vi "Load-default-advanced-params-from-file.vi"(8 "error in":errorcluster, 11 "Data ref. in":refnum<data-value>) -> (0 "error IO":errorcluster, 3 "Data ref.":refnum<data-value>)   [LabVIEW 2013, in "CameraVision.lvlib" / "CV-Main.lvclass"]
doc: "This function loads the default values for the hidden program parameters from an .xml file and writes these values to the parameter groups.\nThe file path for the hidden parameters is '<Application directory>\\Program data\\parameters-hidden.xml'.\nThe hidden parameters can not be changed through the CameraVision program, but can be changed using the 'CV-Set-hidden-parameters.vi' utility."
uses:
  CV-Main.lvclass
  Parameters-advanced.ctl
  Configuration/Configuration-parameters-advanced.ctl
  Acquisition/Acquisition-parameters-advanced.ctl
  Correction/Correction-parameters-advanced.ctl
  Analysis/Analysis-parameters-advanced.ctl
  Temperature/Temperature-parameters-advanced.ctl
  Storage/Storage-parameters-advanced.ctl
  Storage/Storage-types-labels.ctl
  CV-Main.lvclass/CV-Main.ctl
  Read Config params.vi
  Read Acquis params.vi
  Read Storage params.vi
  Read Correct params.vi
  Read Analysis params.vi
  Read Temperature params.vi
  <vilib>/Utility/xml.llb/Read From XML File(string).vi
  Temperature/Overwrite-all-hidden-params.vi
  Analysis/Overwrite-all-hidden-parameters.vi
  Correction/Overwrite-all-hidden-params.vi
  Storage/Overwrite-all-hidden-params.vi
  Acquisition/Overwrite-all-hidden-parameters.vi
  Configuration/Overwrite-all-hidden-params.vi
  Configuration/CV-Configuration.lvclass
  Acquisition/CV-Acquisition.lvclass
  Storage/CV-Storage.lvclass
  Correction/CV-Correction.lvclass
  Analysis/CV-Analysis.lvclass
  Temperature/CV-Temperature.lvclass
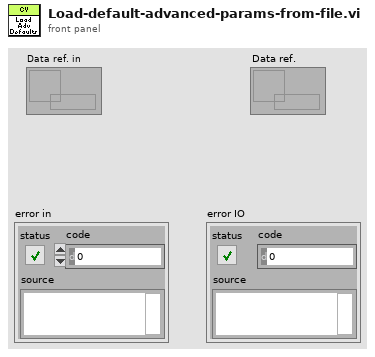
[diagram p1: front panel]
types:
  T1 = typedef "CameraVision.lvlib/CV-Main.lvclass/Parameters-advanced.ctl" = cluster{"Config params adv":T2, "Acquis params adv":T3, "Correct params adv":T4, "Analys params adv":T5, "Temp params adv":T7, "Storage params adv":T8}
  T2 = typedef "CameraVision.lvlib/CV-Configuration.lvclass/Configuration-parameters-advanced.ctl" = cluster{"Image border size":i32, "Framegrabber board":i32, "Framegrabber buffer":i32, "Camera config file":path, "Framegrabber DLL file":path}
  T3 = typedef "CameraVision.lvlib/CV-Acquisition.lvclass/Acquisition-parameters-advanced.ctl" = cluster{"Image acquisition timeout factor":dbl, "Image collection timeout factor":dbl, "Manual trigger ID":u8, "Precision hardware counter":tag, "When to use gate signal?":bool, "Minimum acquisition timeout":i32, "External timing channel":tag, "External gating channel":tag}
  T4 = typedef "CameraVision.lvlib/CV-Correction.lvclass/Correction-parameters-advanced.ctl" = cluster{"2nd image mirror axis":u32, "Cross-correlation decimation":i32, "Cross-correlation algorithm":enum32{"direct", "frequency domain"}, "Always threshold when smoothing?":bool, "Threshold only 2nd camera image?":bool, "Median filter type":cluster{"Order #":i32, "Y Size":i32, "X Size":i32}, "Gaussian filter kernel size":i32, "Gaussian filter kernel number":i32}
  T5 = typedef "CameraVision.lvlib/CV-Analysis.lvclass/Analysis-parameters-advanced.ctl" = cluster{"Melt-pool connectivity":bool, "Melt-pool characteristics":T6[]}
  T6 = typedef "Particle Parameters" = i32
  T7 = typedef "CameraVision.lvlib/CV-Temperature.lvclass/Temperature-parameters-advanced.ctl" = cluster{"Axis origin relative position":dbl, "Regression file relative path":string}
  T8 = typedef "CameraVision.lvlib/CV-Storage.lvclass/Storage-parameters-advanced.ctl" = cluster{"Storage labels":T9, "Characteristics headers":string[], "CharacteristicsTemperature headers":string[]}
  T9 = typedef "CameraVision.lvlib/CV-Storage.lvclass/Storage-types-labels.ctl" = cluster{"Original":string, "Corrected":string, "Binary":string, "Temperature":string, "Characteristics":string, "Mapping":string, "TemperatureValues":string}
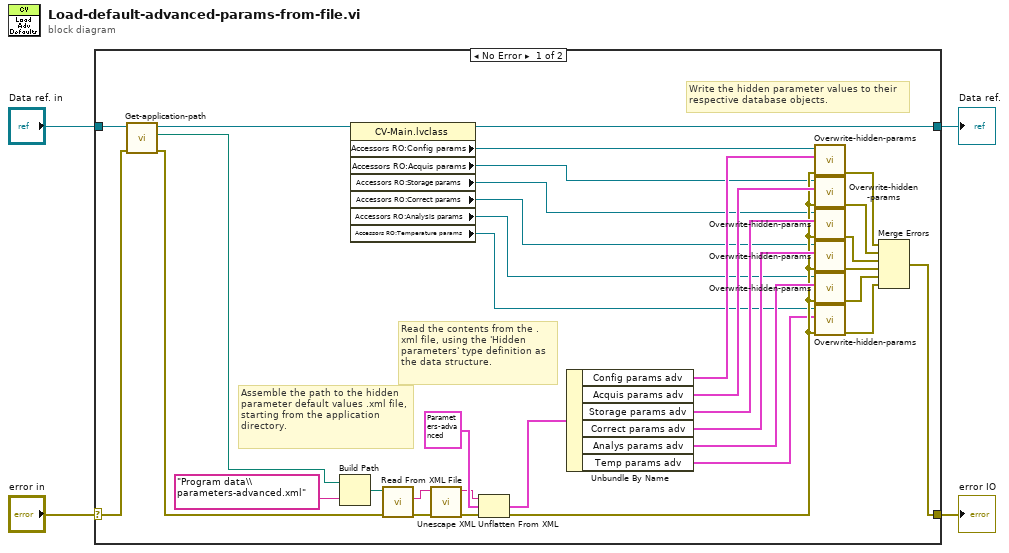
[diagram p0: block diagram]
diagram:
  n1 = case shown="No Error" "error in" {
    selector: "error in" -> [w5 w40]
    tunnel: [w37 w40] -> w4
    tunnel: "Data ref. in" -> [w10 w39]
    tunnel: [w9 w39] -> w1
    frame No Error {
      # "Write the hidden parameter values to their respective database objects."
      # "Read the contents from the .xml file, using the 'Hidden parameters' type definition as the data structure."
      # "Assemble the path to the hidden parameter default values .xml file, starting from the application directory."
      n2 = call "Get-application-path.vi"("error in (no error)"=w5, "Data ref. in"=w10) -> ("error out"=w6:errorcluster, "App path"=w7:path, "Data ref."=w8:refnum<data-value>)  [unwired: 7 in]
      n3 = Build Path(base path=w7, name or relative path="Program data\\parameters-advanced.xml" ("Relative save path")) -> (appended path=w36:path)
      n4 = property class="CV-Main.lvclass"(reference=w8) -> (reference out=w9:refnum<data-value>, "Accessors RO:Config params"=w16:refnum<data-value>, "Accessors RO:Acquis params"=w15:refnum<data-value>, "Accessors RO:Storage params"=w14:refnum<data-value>, "Accessors RO:Correct params"=w13:refnum<data-value>, "Accessors RO:Analysis params"=w12:refnum<data-value>, "Accessors RO:Temperature params"=w11:refnum<data-value>)  [unwired: 1 in, 1 out]
      n5 = call-poly <vilib>:"Read From XML File.vi"("error in (no error)"=w6, "XML File Path"=w36) -> ("error out"=w33:errorcluster, "XML Elements"=w32:string)  [unwired: 7 in, 1 out]
      n6 = call <vilib>:"Unescape XML.vi"("error in (no error)"=w33, "XML String In"=w32) -> ("error out"=w30:errorcluster, "XML String Out"=w31:string)  [unwired: 8 in]
      n7 = Unflatten From XML(xml string=w31, type=T1 {"Config params adv"={"Image border size"=0, "Framegrabber board"=0, "Framegrabber buffer"=0, "Camera config file"=path "", "Framegrabber DLL file"=path ""}, "Acquis params adv"={"Image acquisition timeout factor"=0.0, "Image collection timeout factor"=0.0, "Manual trigger ID"=0, "Precision hardware counter"="", "When to use gate signal?"=FALSE, "Minimum acquisition timeout"=0, "External timing channel"="", "External gating channel"=""}, "Correct params adv"={"2nd image mirror axis"=0, "Cross-correlation decimation"=0, "Cross-correlation algorithm"=enum."direct", "Always threshold when smoothing?"=FALSE, "Threshold only 2nd camera image?"=FALSE, "Median filter type"={"Order #"=0, "Y Size"=0, "X Size"=0}, "Gaussian filter kernel size"=0, "Gaussian filter kernel number"=0}, "Analys params adv"={"Melt-pool connectivity"=FALSE, "Melt-pool characteristics"=[]}, "Temp params adv"={"Axis origin relative position"=0.0, "Regression file relative path"=""}, "Storage params adv"={"Storage labels"={"Original"="", "Corrected"="", "Binary"="", "Temperature"="", "Characteristics"="", "Mapping"="", "TemperatureValues"=""}, "Characteristics headers"=[], "CharacteristicsTemperature headers"=[]}} ("Hidden parameters"), error in (no error)=w30) -> (value=w34:T1, error out=w19:errorcluster)
      n8 = Unbundle By Name(w34) -> ("Config params adv"=w29:T2, "Acquis params adv"=w26:T3, "Storage params adv"=w24:T8, "Correct params adv"=w23:T4, "Analys params adv"=w20:T5, "Temp params adv"=w17:T7)
      n9 = call-poly "Overwrite-hidden-params.vi"("error in (no error)"=w19, "Config params adv"=w29, "Config. params. ref. in"=w16) -> ("error out"=w28:errorcluster)  [unwired: 7 in, 1 out]
      n10 = call-poly "Overwrite-hidden-params.vi"("error in (no error)"=w19, "Acquis params adv"=w26, "Acquis. params. ref. in"=w15) -> ("error out"=w27:errorcluster)  [unwired: 7 in, 1 out]
      n11 = call-poly "Overwrite-hidden-params.vi"("error in (no error)"=w19, "Storage params adv"=w24, "Storage params. ref. in"=w14) -> ("error out"=w25:errorcluster)  [unwired: 7 in, 1 out]
      n12 = call-poly "Overwrite-hidden-params.vi"("error in (no error)"=w19, "Correct params adv"=w23, "Correct. params. ref. in"=w13) -> ("error out"=w22:errorcluster)  [unwired: 7 in, 1 out]
      n13 = call-poly "Overwrite-hidden-params.vi"("error in (no error)"=w19, "Analysis params adv"=w20, "Analysis params. ref. in"=w12) -> ("error out"=w21:errorcluster)  [unwired: 7 in, 1 out]
      n14 = call-poly "Overwrite-hidden-params.vi"("error in (no error)"=w19, "Temp params adv"=w17, "Temp. params. ref. in"=w11) -> ("error out"=w18:errorcluster)  [unwired: 7 in, 1 out]
      n15 = Merge Errors(w28, w27, w25, w22, w21, w18) -> (w37:errorcluster)
    }
    frame Error {
    }
  }
  "error IO" <- w4
  "Data ref." <- w1
